vi "Mobility-Vt-Used Pts_Saturation.vi"(0 "Vg Used":dbl[](array[numeric]), 1 "Length":dbl, 3 "Width":dbl, 5 "Sat Id Used":dbl[](array[numeric]), 9 "Dielectric (d)":dbl, 12 "Dielectric Const":dbl) -> (4 "Mobility":dbl, 6 "Vt":dbl, 10 "Capacitance":dbl, 15 "Threshold Voltage Error":dbl)   [LabVIEW 2015]
uses:
  <vilib>/Analysis/6fits.llb/Confidence Interval (Linear).vi
  <vilib>/Analysis/NI_AALPro.lvlib
panel:
  out "delta slope":dbl
  out "delta intercept":dbl
  out "residue":dbl
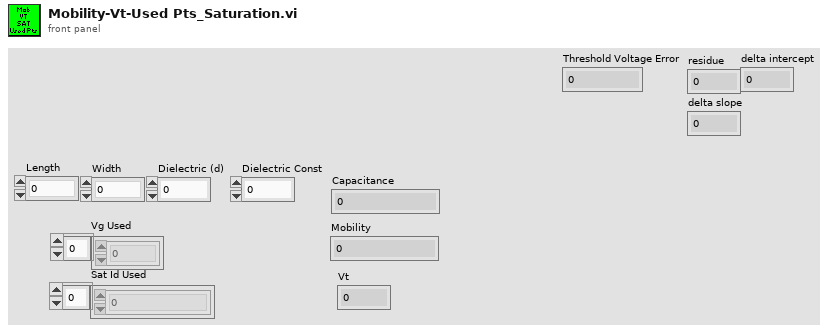
[diagram p1: front panel]
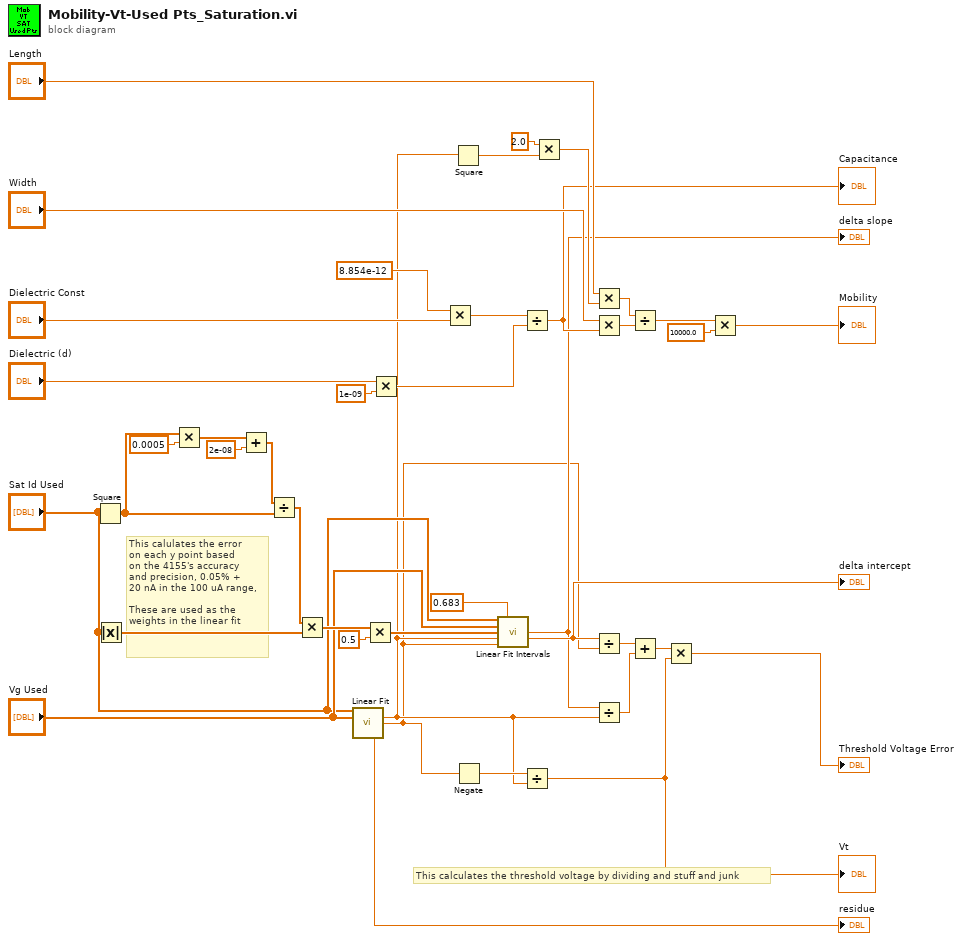
[diagram p0: block diagram]
diagram:
  # "This calulates the error \non each y point based\non the 4155's accuracy\nand precision, 0.05% + \n20 nA in the 100 uA range,\n\nThese are used as the \nweights in the linear fit"
  # "This calculates the threshold voltage by dividing and stuff and junk"
  n1 = Square(x="Sat Id Used") -> (x^2=w11:dbl[])
  n2 = Absolute Value(x="Sat Id Used") -> (abs(x)=w15:dbl[])
  n3 = Multiply(x=w11, y=0.0005) -> (x*y=w23:dbl[])
  n4 = Add(x=w23, y=2e-08) -> (x+y=w21:dbl[])
  n5 = Divide(x=w21, y=w11) -> (x/y=w20:dbl[])
  n6 = Multiply(x=w20, y=w15) -> (x*y=w19:dbl[])
  n7 = call <vilib>:"Linear Fit.vi"("Y"="Sat Id Used", "X"="Vg Used") -> ("slope"=w5:dbl, "intercept"=w4:dbl, "residue"=→"residue":dbl)  [unwired: 9 in, 2 out]
  n8 = Multiply(x=w19, y=0.5) -> (x*y=w10:dbl[])
  n9 = Multiply(x="Dielectric (d)", y=1e-09) -> (x*y=w40:dbl)
  n10 = Multiply(x=8.854e-12, y="Dielectric Const") -> (x*y=w41:dbl)
  n11 = Square(x=w5) -> (x^2=w16:dbl)
  n12 = Negate(x=w4) -> (-x=w27:dbl)
  n13 = call-poly <vilib>:"Linear Fit Intervals.vi"("Y"="Sat Id Used", "confidence level"=0.683, "X"="Vg Used", "Weight"=w10, "slope"=w5, "intercept"=w4) -> ("delta slope"=w6:dbl, "delta intercept"=w7:dbl)  [unwired: 5 in, 3 out]
  "delta intercept" <- w7
  "delta slope" <- w6
  n14 = Divide(x=w41, y=w40) -> (x/y=w26:dbl)
  "Capacitance" <- w26
  n15 = Divide(x=w27, y=w5) -> (x/y=w2:dbl)
  "Vt" <- w2
  n16 = Multiply(x=2.0, y=w16) -> (x*y=w34:dbl)
  n17 = Multiply(x="Length", y=w34) -> (x*y=w33:dbl)
  n18 = Multiply(x="Width", y=w26) -> (x*y=w32:dbl)
  n19 = Divide(x=w7, y=w4) -> (x/y=w9:dbl)
  n20 = Divide(x=w6, y=w5) -> (x/y=w8:dbl)
  n21 = Divide(x=w33, y=w32) -> (x/y=w30:dbl)
  n22 = Add(x=w9, y=w8) -> (x+y=w3:dbl)
  n23 = Multiply(x=w3, y=w2) -> (x*y=→"Threshold Voltage Error":dbl)
  n24 = Multiply(x=w30, y=10000.0) -> (x*y=→"Mobility":dbl)
